vi "Get All Drives Info.vi"() -> (3 "Drives Information":T1(array[cluster]) {"VolumeSerialNumber" format="%.0x"})   [LabVIEW 2011]
doc: "An example of using the drive information VI's.\nThe VI first bulds alist of all available drives, then iterates through each one getting identifiers, cluster and space information about that drive."
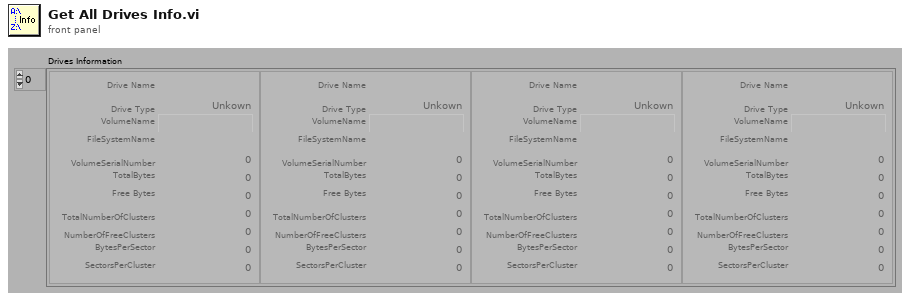
[diagram p1: front panel]
types:
  T1 = cluster{"Drive Name":string, "Drive Type":enum16{"Unkown", "No Root", "Removable", "Fixed", "Remote", "CD Rom", "Ramdisk"}, "VolumeName":string, "FileSystemName":string, "VolumeSerialNumber":u32, "TotalBytes":u32, "Free Bytes":u32, "TotalNumberOfClusters":u32, "NumberOfFreeClusters":u32, "BytesPerSector":u32, "SectorsPerCluster":u32}[]
  T2 = enum16{"Unkown", "No Root", "Removable", "Fixed", "Remote", "CD Rom", "Ramdisk"}
  T3 = cluster{"string":string, "Drive Type":enum16{"Unkown", "No Root", "Removable", "Fixed", "Remote", "CD Rom", "Ramdisk"}, "VolumeName":string, "FileSystemName":string, "VolumeSerialNumber":u32, "TotalBytes":u32, "Free Bytes":u32, "TotalNumberOfClusters":u32, "NumberOfFreeClusters":u32, "BytesPerSector":u32, "SectorsPerCluster":u32}
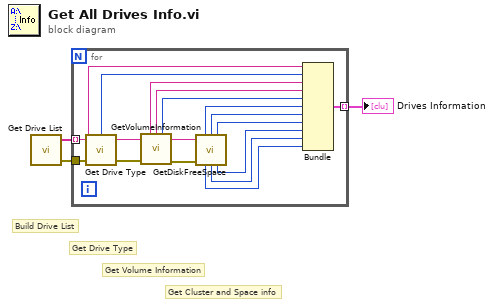
[diagram p0: block diagram]
diagram:
  # "Get Cluster and Space info"
  # "Get Volume Information"
  # "Get Drive Type"
  # "Build Drive List"
  n1 = call "Get Drive List.vi"() -> ("Drive List"=w3:string[], "error out"=w2:errorcluster)  [unwired: 1 in]
  n2 = for {
    tunnel: w3 -> [w15] mode=indexing
    tunnel: w2 -> [w20]
    tunnel: [w4] -> w1 mode=indexing
    n3 = call "Get Drive Type.vi"("error in (no error)"=w20, "Root Path name (C:\\)"=w15) -> ("error out"=w19:errorcluster, "Dup Root Path name (C:\\)"=w17:string, "Drive Type"=w14:T2)  [unwired: 1 out]
    n4 = call "GetVolumeInformation.vi"("RootPathName (C:\\)"=w17, "error in (no error)"=w19) -> ("VolumeName"=w13:string, "FileSystemName"=w12:string, "VolumeSerialNumber"=w11:u32, "Dup Root Path name (C:\\)"=w16:string, "error out"=w18:errorcluster)  [unwired: 9 out]
    n5 = call "GetDiskFreeSpace.vi"("RootPathName (C:\\)"=w16, "error in (no error)"=w18) -> ("TotalBytes"=w10:u32, "Free Bytes"=w9:u32, "TotalNumberOfClusters"=w8:u32, "SectorsPerCluster"=w5:u32, "BytesPerSector"=w6:u32, "NumberOfFreeClusters"=w7:u32)  [unwired: 8 out]
    n6 = Bundle("string"=w15, "Drive Type"=w14, "VolumeName"=w13, "FileSystemName"=w12, "VolumeSerialNumber"=w11, "TotalBytes"=w10, "Free Bytes"=w9, "TotalNumberOfClusters"=w8, "NumberOfFreeClusters"=w7, "BytesPerSector"=w6, "SectorsPerCluster"=w5) -> (w4:T3)  [unwired: 1 out]
  }
  "Drives Information" <- w1
